vi "Test IntegrationShellTest.vi"(8 "error in (no error)":errorcluster, 11 "TestCase in":refnum<class "CarWashTestCases.lvclass">) -> (0 "error out":errorcluster, 3 "TestCase out":refnum<class "CarWashTestCases.lvclass">)   [LabVIEW 2018, in "CarWashTestCases.lvclass"]
uses:
  CarWashTestCases.lvclass
  <vilib>/addons/_JKI Toolkits/VI Tester/TestCase.llb/TestCase.lvclass
  C:/Program Files/National Instruments/LabVIEW 2018/vi.lib/addons/_JKI Toolkits/VI Tester/TestCase.llb/TestCase.lvclass
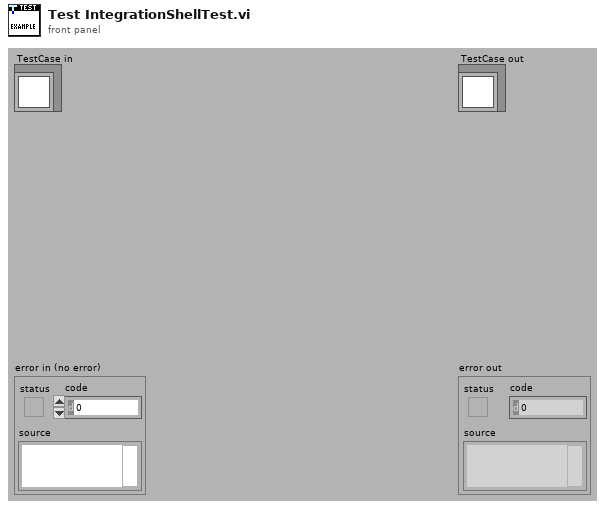
[diagram p1: front panel]
types:
  T1 = enum32{"Bad", "Idle", "Run top level", "Running"}
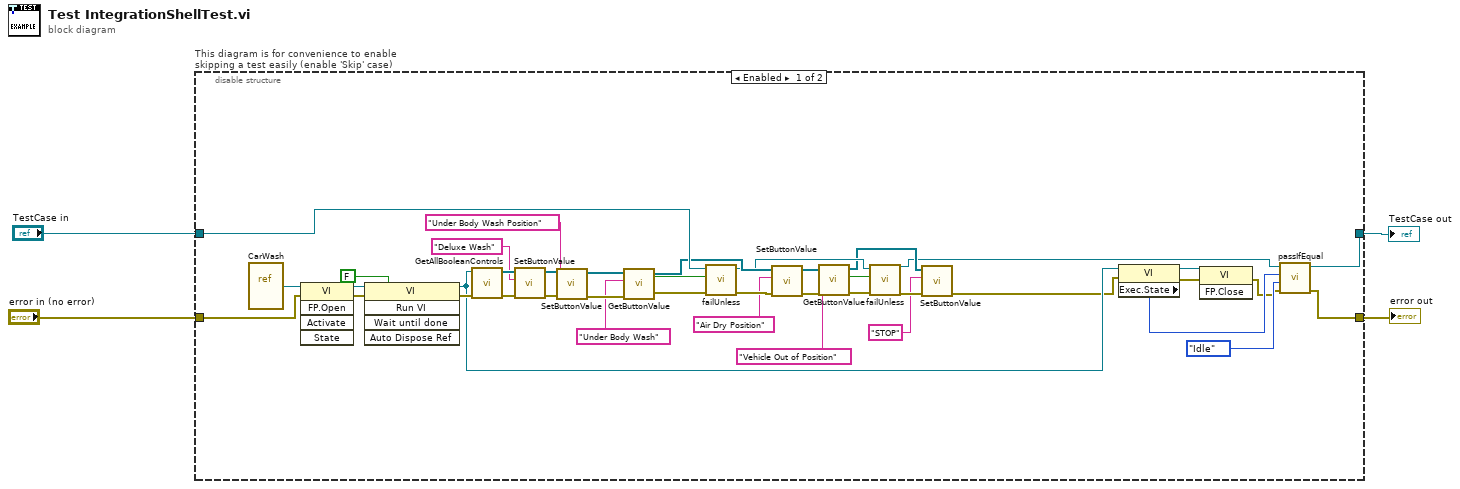
[diagram p0: block diagram]
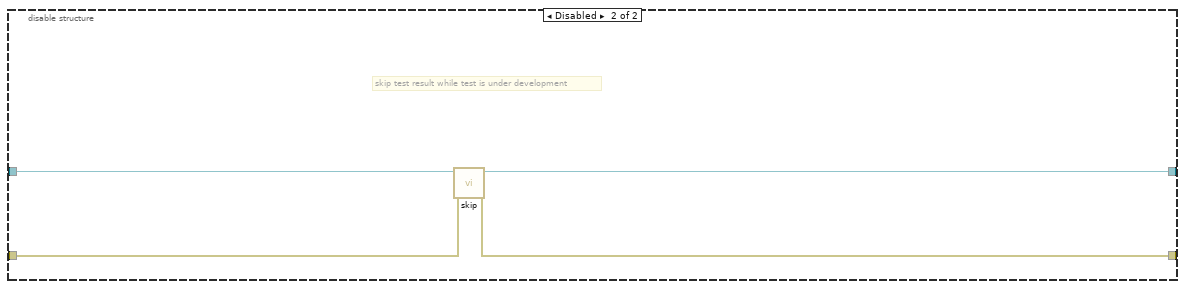
[diagram p2: hidden frame]
diagram:
  n1 = disable-structure "This diagram is for convenience to enable skipping a test easily (enable 'Skip' case)" shown="Enabled" {
    disable-tunnel: "TestCase in" -> [w30 w48]
    disable-tunnel: [w12 w46] -> w1
    disable-tunnel: [w11 w47] -> w3
    disable-tunnel: "error in (no error)" -> [w37 w45]
    frame Enabled {
      n2 = vi-ref "CarWash.vi"() -> (w38:refnum<vi>)
      n3 = invoke class="VI" method="FP.Open"(reference=w38, error in=w37) -> (reference out=w41:refnum<vi>, error out=w40:errorcluster)  [unwired: 3 in, 3 out]
      n4 = invoke class="VI" method="Run VI"(reference=w41, error in=w40, "Wait until done"=FALSE ("Wait Until Done")) -> (reference out=w14:refnum<vi>, error out=w39:errorcluster)  [unwired: 2 in, 3 out]
      n5 = call "GetAllBooleanControls.vi"("error in (no error)"=w39, "VI in"=w14) -> ("error out"=w42:errorcluster, "Boolean Controls"=w44:refnum<vi>[])  [unwired: 8 in]
      n6 = call "SetButtonValue.vi"("error in (no error)"=w42, "label"="Deluxe Wash" ("y"), "Buttons"=w44) -> ("error out"=w36:errorcluster, "Buttons out"=w35:refnum<vi>[])  [unwired: 7 in]
      n7 = call "SetButtonValue.vi"("error in (no error)"=w36, "label"="Under Body Wash Position", "Buttons"=w35) -> ("error out"=w34:errorcluster, "Buttons out"=w33:refnum<vi>[])  [unwired: 7 in]
      n8 = call "GetButtonValue.vi"("error in (no error)"=w34, "label"="Under Body Wash", "Buttons"=w33) -> ("error out"=w29:errorcluster, "Value"=w28:bool, "Buttons out"=w25:refnum<vi>[])  [unwired: 6 in]
      n9 = call-dynamic "failUnless.vi"("error in (no error)"=w29, "pass"=w28, "TestCase in"=w30) -> ("error out"=w26:errorcluster, "TestCase out"=w18:refnum<class "CarWashTestCases.lvclass">)  [unwired: 7 in]
      n10 = call "SetButtonValue.vi"("error in (no error)"=w26, "label"="Air Dry Position", "Buttons"=w25) -> ("error out"=w23:errorcluster, "Buttons out"=w22:refnum<vi>[])  [unwired: 7 in]
      n11 = call "GetButtonValue.vi"("error in (no error)"=w23, "label"="Vehicle Out of Position", "Buttons"=w22) -> ("error out"=w20:errorcluster, "Value"=w19:bool, "Buttons out"=w17:refnum<vi>[])  [unwired: 6 in]
      n12 = call-dynamic "failUnless.vi"("error in (no error)"=w20, "pass"=w19, "TestCase in"=w18) -> ("error out"=w16:errorcluster, "TestCase out"=w13:refnum<class "CarWashTestCases.lvclass">)  [unwired: 7 in]
      n13 = call "SetButtonValue.vi"("error in (no error)"=w16, "label"="STOP", "Buttons"=w17) -> ("error out"=w5:errorcluster)  [unwired: 7 in, 1 out]
      n14 = property class="VI"(reference=w14, error in=w5) -> (reference out=w8:refnum<vi>, error out=w7:errorcluster, "Exec.State"=w9:T1)
      n15 = invoke class="VI" method="FP.Close"(reference=w8, error in=w7) -> (error out=w6:errorcluster)  [unwired: 1 in, 2 out]
      n16 = call-dynamic "passIfEqual.vi"("error in (no error)"=w6, "y"=T1."Idle", "x"=w9, "TestCase in"=w13) -> ("error out"=w11:errorcluster, "TestCase out"=w12:refnum<class "CarWashTestCases.lvclass">)  [unwired: 6 in]
    }
    frame Disabled {
      # "skip test result while test is under development"
      n17 = call <vilib>:"skip.vi"("error in (no error)"=w45, "TestCase in"=w48) -> ("error out"=w47:errorcluster, "TestCase out"=w46:refnum<class "CarWashTestCases.lvclass">)  [unwired: 8 in]
    }
  }
  "error out" <- w3
  "TestCase out" <- w1
